vi "rad_Write Deployment Results to File.vi"(8 "error in":errorcluster, 9 "App Image Path":path, 10 "Targets Deployment":string[][](array[string]), 11 "Targets":T1[](array[typedef]) {"Primary NIC"."IP Address Request Mode" items=["Static"=1, "DHCP/Link-Local"=2, "Link-Local Only"=4, "DHCP Only"=8]}) -> (0 "error out":errorcluster)   [LabVIEW 2023]
uses:
  Targets/TypeDefs/rad_Target Information.ctl
  Targets/TypeDefs/rad_Target Network Settings.ctl
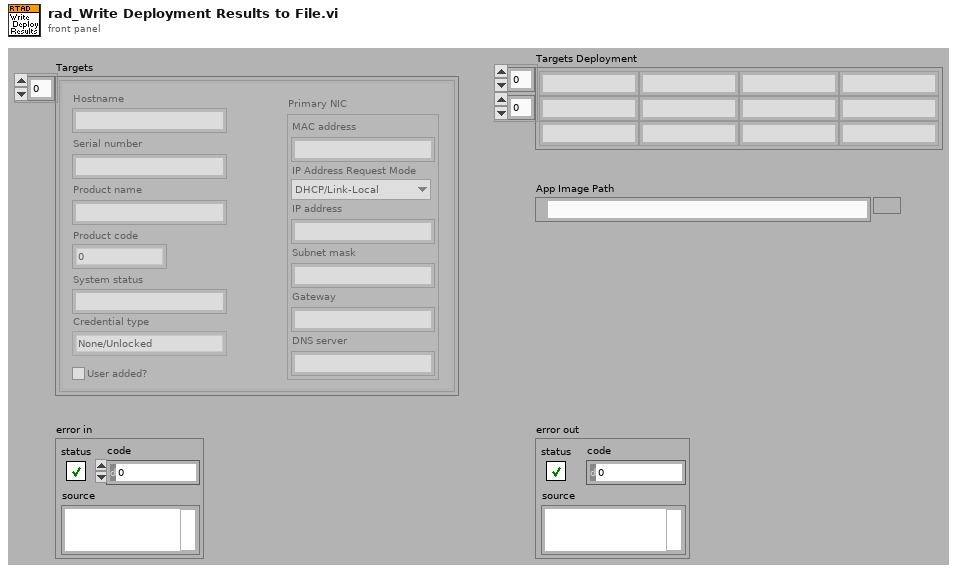
[diagram p1: front panel]
types:
  T1 = typedef "rad_Target Information.ctl" = cluster{"Hostname":string, "Serial number":string, "Product name":string, "Product code":i32, "System status":string, "Credential type":enum16{"None/Unlocked", "FTP Password", "NIAuth Credentials"}, "User added?":bool, "Primary NIC":T2}
  T2 = typedef "rad_Target Network Settings.ctl" = cluster{"MAC address":string, "IP Address Request Mode":i32, "IP address":string, "Subnet mask":string, "Gateway":string, "DNS server":string}
  T3 = enum16{"open", "replace", "create", "open or create", "replace or create", "replace or create with confirmation"}
  T4 = typedef "rad_Application Image Properties.ctl" = cluster{"Name":string, "Version":string, "Time":timestamp, "Description":string, "Key":string, "Chassis":string, "FPGA Properties":T5, "Model":string, "Retrieve":string[], "Deploy":string[], "Installed Software":string[]}
  T5 = typedef "rad_FPGA Properties.ctl" = T6[]
  T6 = typedef "rad_FPGA Flash Properties.ctl" = cluster{"Resource Name":string, "Path":path}
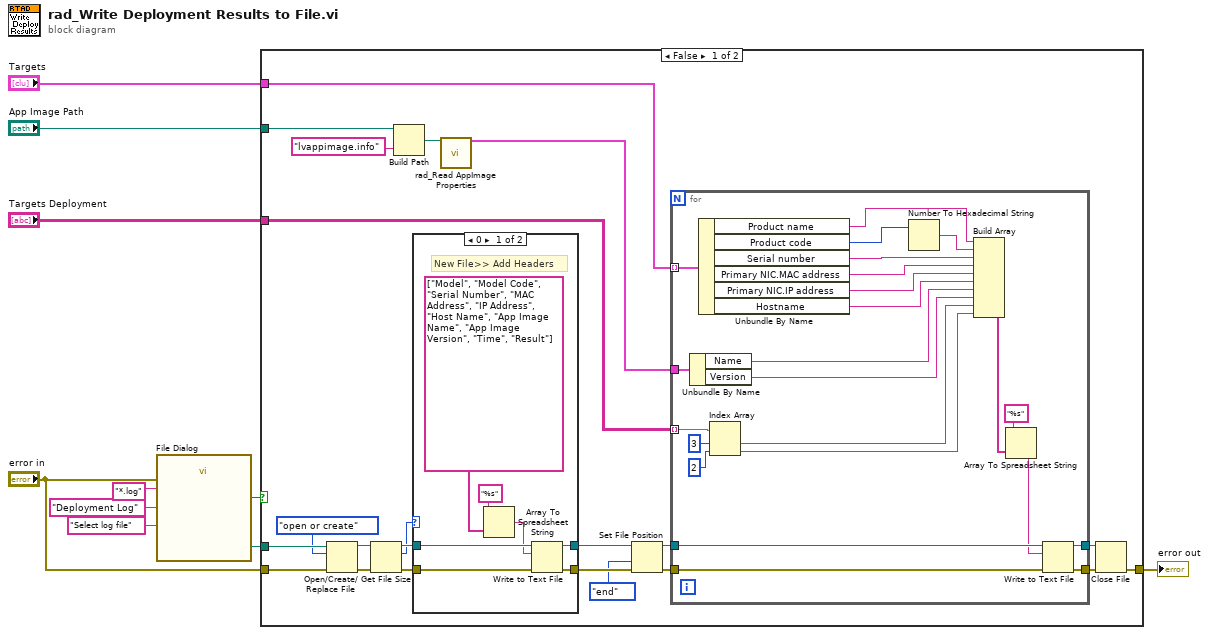
[diagram p0: block diagram]
diagram:
  n1 = call "File Dialog"("prompt"="Select log file", "error in"="error in", "pattern (all files)"="*.log", "pattern label"="Deployment Log") -> ("selected path"=w6:path, "cancelled"=w7:bool)  [unwired: 3 in, 7 out]
  n2 = case shown="False" w7 {
    tunnel: w6 -> [w32 _]
    tunnel: "error in" -> [w31 w65]
    tunnel: "Targets" -> [w30 _]
    tunnel: "Targets Deployment" -> [w29 _]
    tunnel: [w26 w65] -> w3
    tunnel: "App Image Path" -> [w14 _]
    frame False {
      n3 = Open/Create/Replace File(file path (use dialog)=w32, error in=w31, operation (0:open)=T3."open or create") -> (refnum out=w24:refnum<file>, error out=w23:errorcluster)  [unwired: 4 out]
      n4 = Get File Size(file=w24, error in=w23) -> (refnum out=w19:refnum<file>, size (in bytes)=w18:i64, 0:w20:errorcluster)
      n5 = Build Path(base path=w14, name or relative path="lvappimage.info") -> (appended path=w12:path)
      n6 = case shown="0" w18 {
        tunnel: w20 -> [w36 w40]
        tunnel: w19 -> [w37 w41]
        tunnel: [w39 w40] -> w17
        tunnel: [w38 w41] -> w16
        frame 0 {
          # "New File>> Add Headers"
          n7 = Array To Spreadsheet String(array=string[] ["Model", "Model Code", "Serial Number", "MAC Address", "IP Address", "Host Name", "App Image Name", "App Image Version", "Time", "Result"], 3:"%s" ("format string")) -> (spreadsheet string=w33:string)  [unwired: 1 out]
          n8 = Write to Text File(file (use dialog)=w37, text=w33, error in=w36) -> (refnum out=w38:refnum<file>, error out=w39:errorcluster)  [unwired: 2 out]
        }
        frame Default {
        }
      }
      n9 = call "rad_Read AppImage Properties.vi"("AppImage Properties Path"=w12) -> ("AppImage Properties"=w11:T4)  [unwired: 13 in, 5 out]
      n10 = Set File Position(refnum=w16, from (0:start)=enum16{"start", "end", "current"}."end", error in=w17) -> (refnum out=w22:refnum<file>, error out=w21:errorcluster)  [unwired: 1 out]
      n11 = for {
        tunnel: w22 -> [w58]
        tunnel: w30 -> [w64] mode=indexing
        tunnel: w29 -> [w63] mode=indexing
        tunnel: w21 -> [w56]
        tunnel: [w55] -> w27
        tunnel: [w54] -> w28
        tunnel: w11 -> [w50]
        n12 = Unbundle By Name(w50) -> ("Name"=w49:string, "Version"=w48:string)
        n13 = Unbundle By Name(w64) -> ("Product name"=w62:string, "Product code"=w43:i32, "Serial number"=w44:string, "Primary NIC.MAC address"=w45:string, "Primary NIC.IP address"=w61:string, "Hostname"=w60:string)
        n14 = Index Array(array=w63, index #1=3 ("index"), index #2=2 ("index")) -> (element #1=w52:string, element #2=w47:string)
        n15 = Number To Hexadecimal String(2:w43) -> (0:w42:string)  [unwired: 1 in]
        n16 = Build Array(w62, w42, w44, w45, w61, w60, w49, w48, w52, w47) -> (w59:string[])
        n17 = Array To Spreadsheet String(array=w59, 3:"%s" ("format string")) -> (spreadsheet string=w57:string)  [unwired: 1 out]
        n18 = Write to Text File(file (use dialog)=w58, text=w57, error in=w56) -> (refnum out=w55:refnum<file>, error out=w54:errorcluster)  [unwired: 2 out]
      }
      n19 = Close File(refnum=w27, error in=w28) -> (error out=w26:errorcluster)  [unwired: 1 out]
    }
    frame True {
    }
  }
  "error out" <- w3
